vi "setColor.vi"(8 "error in (no error)":errorcluster, 10 "Color Box":u32(colorbox), 11 "junkClass01 in":refnum<class "junkClass01.lvclass">) -> (0 "error out":errorcluster, 3 "junkClass01 out":refnum<class "junkClass01.lvclass">)   [LabVIEW 2013, in "junkClass01.lvclass"]
uses:
  junkClass01.lvclass
  junkClass01.lvclass/junkClass01.ctl
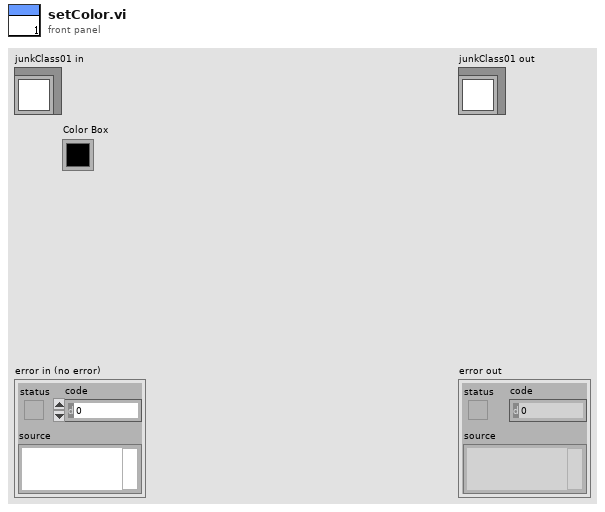
[diagram p1: front panel]
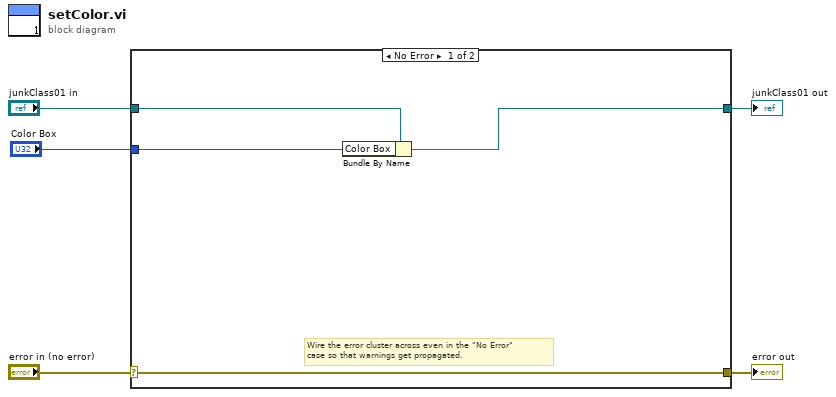
[diagram p0: block diagram]
diagram:
  n1 = case shown="No Error" "error in (no error)" {
    selector: "error in (no error)" -> [w9 w11]
    tunnel: [w9 w11] -> w4
    tunnel: [w7 w10] -> w2
    tunnel: "junkClass01 in" -> [w8 w10]
    tunnel: "Color Box" -> [w6 _]
    frame No Error {
      # "Wire the error cluster across even in the \"No Error\"\ncase so that warnings get propagated."
      n2 = Bundle By Name(cluster=w8, "Color Box"=w6) -> (w7:refnum<class "junkClass01.lvclass">)
    }
    frame Error {
    }
  }
  "error out" <- w4
  "junkClass01 out" <- w2
